vi "Rising&Falling.vi"(11 "input":bool) -> (2 "Falling":bool, 3 "Rising":bool)   [LabVIEW 2014]
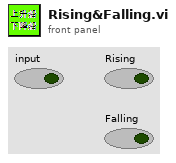
[diagram p1: front panel]
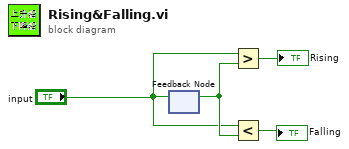
[diagram p0: block diagram]
diagram:
  n1 = feedback #1() -> (w3:bool)  [unwired: 1 in]
  n2 = feedback-in #1("input") -> ()
  n3 = Greater?(x="input", y=w3) -> (0:→"Rising":bool)
  n4 = Less?(x="input", y=w3) -> (x < y?=→"Falling":bool)
